vi "Undefined State Error Popup.vi"(9 "String":string, 11 "This VI (Caller if unwired)":refnum<vi>) -> ()   [LabVIEW 2013, in "State Machine Lib.lvlib"]
doc: "Alerts the user that an undefined state has been reached. Dialog with the offending vi and state pops-up."
uses:
  State Machine Lib.lvlib
panel:
  out "error out":errorcluster
  in  "error in":errorcluster
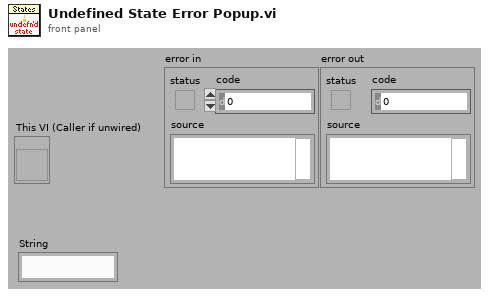
[diagram p1: front panel]
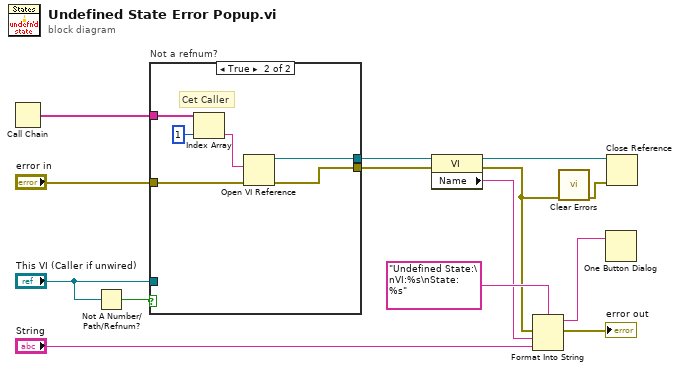
[diagram p0: block diagram]
diagram:
  n1 = Call Chain() -> (call chain=w4:string[])
  n2 = Not A Number/Path/Refnum?(number/path/refnum="This VI (Caller if unwired)") -> (NaN/Path/Refnum?=w9:bool)
  n3 = case "Not a refnum?" shown="True" w9 {
    tunnel: "This VI (Caller if unwired)" -> [w16 _]
    tunnel: [w16 w17] -> w7
    tunnel: "error in" -> [w15 w19]
    tunnel: [w15 w18] -> w5
    tunnel: w4 -> [_ w22]
    frame False {
    }
    frame True {
      # "Cet Caller"
      n4 = Index Array(array=w22, index=1) -> (element=w20:string)
      n5 = Open VI Reference(vi path=w20, error in (no error)=w19) -> (vi reference=w17:refnum<vi>, error out=w18:errorcluster)  [unwired: 4 out]
    }
  }
  n6 = property class="VI"(reference=w7, error in=w5) -> (reference out=w3:refnum<vi>, error out=w2:errorcluster, "Name"=w13:string)
  n7 = Format Into String(format string="Undefined State:\nVI:%s\nState: %s", error in=w2, w13, "String") -> (resulting string=w11:string, error out=→"error out":errorcluster)  [unwired: 1 in]
  n8 = call <vilib>:"Clear Errors.vi"("error in (no error)"=w2) -> ("error out"=w1:errorcluster)  [unwired: 6 out]
  n9 = One Button Dialog(message=w11) -> ()  [unwired: 2 out]
  n10 = Close Reference(reference=w3, error in (no error)=w1) -> ()  [unwired: 1 out]
